vi "SlopeFitFromCSV.vi"() -> ()   [LabVIEW 2016]
uses:
  <vilib>/Utility/file.llb/Read Delimited Spreadsheet (DBL).vi
  <vilib>/Analysis/NI_AALPro.lvlib
panel:
  out "R-square":dbl
  out "XY Graph":cluster{dbl[], "Best Linear Fit":dbl[]}[](graph)
  out "slope":dbl
  out "intercept":dbl
  out "all rows":dbl[][](array[numeric])
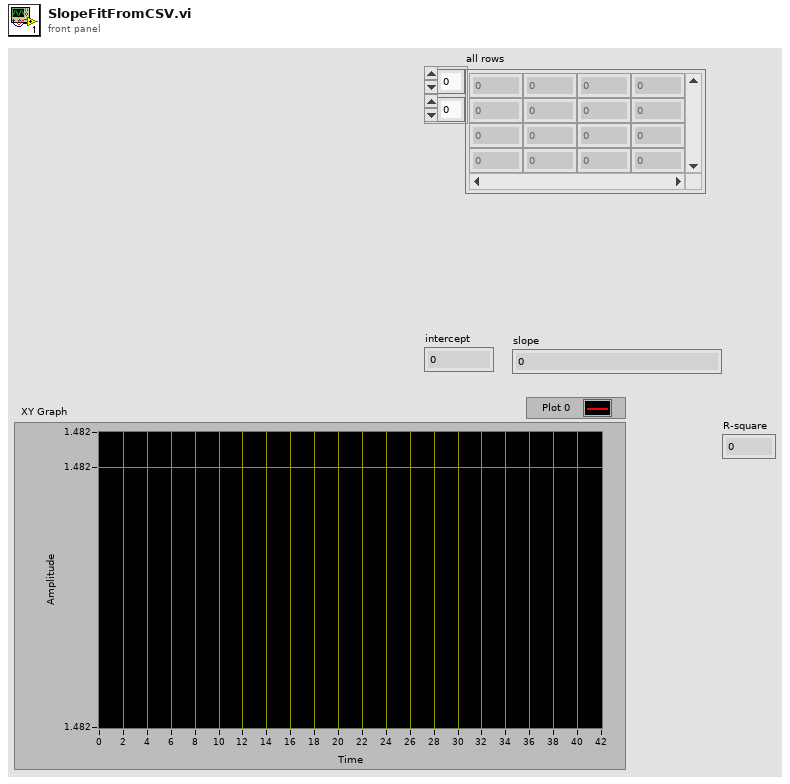
[diagram p1: front panel]
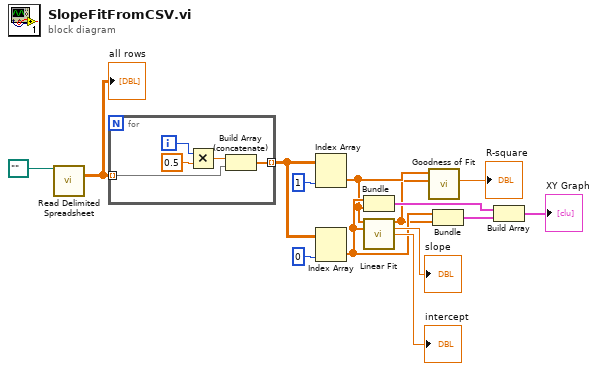
[diagram p0: block diagram]
diagram:
  n1 = call-poly <vilib>:"Read Delimited Spreadsheet.vi"("file path (dialog if empty)"=path "") -> ("all rows"=w13:dbl[][])  [unwired: 9 in, 5 out]
  "all rows" <- w13
  n2 = for {
    tunnel: w13 -> [w19] mode=indexing
    tunnel: [w15] -> w12 mode=indexing
    i -> [w17]
    n3 = Multiply(x=w17, y=0.5) -> (x*y=w18:dbl)
    n4 = Build Array (concatenate)(w18, w19) -> (w15:dbl[])
  }
  n5 = Index Array(array=w12, index (col)=1 ("disabled index (col)")) -> (element=w3:dbl[])  [unwired: 1 in]
  n6 = Index Array(array=w12, index (col)=0 ("disabled index (col)")) -> (element=w7:dbl[])  [unwired: 1 in]
  n7 = Bundle(w7, w3) -> (w6:cluster{dbl[], dbl[]})  [unwired: 1 in]
  n8 = call <vilib>:"Linear Fit.vi"("Y"=w3, "X"=w7) -> ("Best Linear Fit"=w2:dbl[], "slope"=→"slope":dbl, "intercept"=→"intercept":dbl)  [unwired: 9 in, 2 out]
  n9 = call <vilib>:"Goodness of Fit.vi"("Best Fit"=w2, "Y"=w3) -> ("R-square"=→"R-square":dbl)  [unwired: 6 in, 3 out]
  n10 = Bundle(w7, "Best Linear Fit"=w2) -> (w5:cluster{dbl[], "Best Linear Fit":dbl[]})  [unwired: 1 in]
  n11 = Build Array(w6, w5) -> (→"XY Graph":cluster{dbl[], "Best Linear Fit":dbl[]}[])
